vi "ISEG_HVChannel.ProcCases.vi"(0 "i ref in":refnum<vi>, 1 "selector":string, 2 "Data":T1, 3 "call cluster":T2={"Object"="", "Selector"="", "CallType"=enum."synchronous", "Async Object"="", "Async Selector"="", "Data Descriptor"="", "Data"=[], "Error #"=0, "Expire"=0}, 5 "error in (no error)":errorcluster) -> (14 "i ref out":refnum<vi>, 17 "answer cluster":T2={"Object"="", "Selector"="", "CallType"=enum."synchronous", "Async Object"="", "Async Selector"="", "Data Descriptor"="", "Data"=[], "Error #"=0, "Expire"=0}, 19 "error out":errorcluster)   [LabVIEW 2014, in "ISEG_HVChannel.lvlib"]
doc: "This method is called by a process from within the default case in the event loop. The methods of a class that are linked to events will be called from THIS method. Add your code here."
uses:
  ISEG_HVChannel.lvlib
  CS_Core/CSSystem/CoreDefs/CoreDefs.call_type.ctl
  CS_Core/BaseProcess/BaseProcess.descriptor string definition.ctl
  CS_Core/CSSystem/CoreDefs/CoreDefs.rawDataType.ctl
  CS_Core/CSApplicationBaseClasses/PSChannelBase/PSChannelBase.serviceType.ctl
  CS_Core/CSApplicationBaseClasses/PSChannelBase/PSChannelBase.directionType.ctl
  CSlibraries/UtilityLib/UtilityLib.valueStatus.ctl
  CS_Core/CSSystem/CoreDefs/CoreDefs.error_type.ctl
  CS_Core/CSSystem/CoreDefs/CoreDefs.error_severity.ctl
  CS_Core/CSSystem/CoreLib/CoreLib.string 2 byte array.vi
  CS_Core/CSSystem/CoreLib/CoreLib.byte array 2 int.vi
  CS_Core/CSSystem/CoreLib/CoreLib.byte array 2 double.vi
  CS_Core/CSSystem/CoreLib/CoreLib.double 2 byte array.vi
  CS_Core/CSSystem/CoreLib/CoreLib.short 2 byte array.vi
  CS_Core/CSSystem/CoreLib/CoreLib.byte array 2 short.vi
  CS_Core/CSSystem/CoreLib/CoreLib.lvlib
  CS_Core/BaseProcess/BaseProcess.lvlib
  CS_Core/CSApplicationBaseClasses/PSChannelBase/PSChannelBase.lvlib
  CSlibraries/UtilityLib/UtilityLib.lvlib
  CS_Core/CAEObj/CAEObj.lvlib
  CS_Core/CSApplicationBaseClasses/DeviceBase/DeviceBase.lvlib
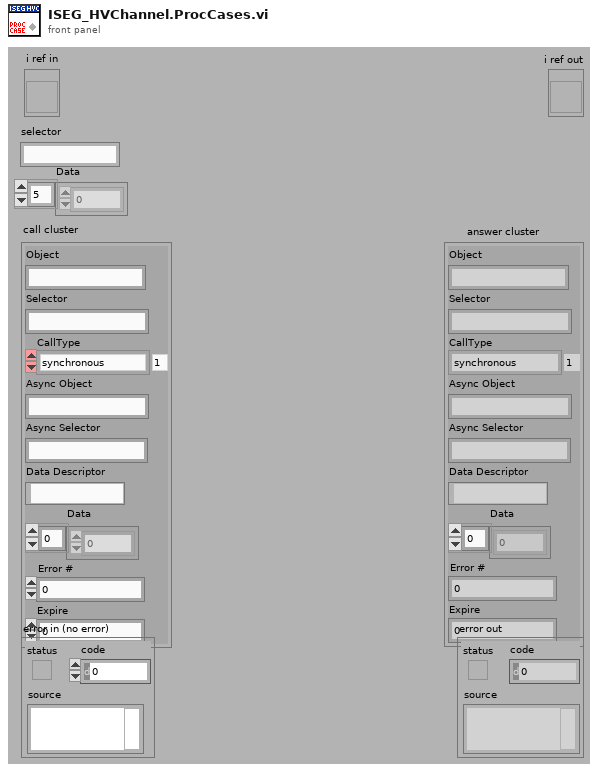
[diagram p1: front panel]
types:
  T1 = typedef "CoreDefs.rawDataType.ctl" = i8[]
  T2 = typedef "CoreDefs.call_type.ctl" = cluster{"Object":string, "Selector":string, "CallType":enum16{"simple", "synchronous", "asynchronous"}, "Async Object":string, "Async Selector":string, "Data Descriptor":T3, "Data":T1, "Error #":i32, "Expire":u32}
  T3 = typedef "BaseProcess.lvlib/BaseProcess.descriptor string definition.ctl" = string
  T4 = typedef "UtilityLib.lvlib/UtilityLib.valueStatus.ctl" = enum16{"no info available", "stand by/off", "on", "warning", "alarm/malfunction", "not implemented", "user action required", "important information", "system default", "control default", "indicator default", "button default"}
  T5 = typedef "PSChannelBase.lvlib/PSChannelBase.directionType.ctl" = enum16{"unknown", "update actual value", "update nominal value", "update both"}
  T6 = typedef "PSChannelBase.lvlib/PSChannelBase.serviceType.ctl" = enum16{"onOff", "voltage", "current", "tripCurrent", "rampUpSpeed", "rampDownSpeed", "status"}
  T7 = typedef "CoreDefs.error_severity.ctl" = enum16{"undefined", "information", "warning", "error", "fatal"}
  T8 = typedef "CoreDefs.error_type.ctl" = enum16{"no error", "can't load process", "can't unload process", "process does not exist", "can't install process", "can't remove process", "unknown function", "time out", "can't execute function", "duplicate queue name", "super not found", "caller queue invalid", "can't ping process", "unknown error", "VISA Error", "VISA timeout", "GPIB timeout", "GPIB error", "communication error", "data type mismatch", "can't read data from OPC server", "can't write data to OPC server", "OET error", "function not implemented", "process already exists", "invalid Shared Variable name", "error writing Shared Variable", "error reading Shared Variable", "invalid client name", "corrupt database", "unknown class", "call not authorized", "parameter out of range", "OET timeout: can't get data to modify", "invalid queue name", "requested operation incompatible with current state", "event undefined", "event disabled", "state undefined", "caller is not a friend", "EventBuilder: bad eventID", "EventBuilder: no DAQ devices", "a thread must not stop itself", "UNUSED ELEMENT4", "DiscArchiver: eventData incomplete", "DiscArchiver: eventData does not belong to run", "DiscArchiver: can't open file", "DiscArchiver: can't write to file", "DiscArchiver: available disc space low", "can't acquire semaphore", "error reading data from database", "notifier object is not existing", "can't register process", "can't unregister process", "illegal event type", "object disabled", "object already exists", "can't change state", "Instrument not found", "no connection to remote node", "invalid reference", "N/A", "UNUSED ELEMENT 1", "element not found", "illegal TCP/IP connection detected", "object does not exist", "invalid access ID", "unknown CS system", "invalid privilige", "unsupported data type", "unsupported server type", "IO server already exists", "Shared Variable already exists"}
  T9 = typedef "PSChannelBase.lvlib/PSChannelBase.i attribute.ctl" = cluster{"defaultChannelIndex":i32, "nofChannels":i32, "defaultChannelIndexID":i32, "nofChannelsID":i32, "actValues":T10, "nomValues":T10, "logicalName":string[], "physicalName":string[], "logicalNameID":i32, "physicalNameID":i32}
  T10 = typedef "PSChannelBase.lvlib/PSChannelBase.parameters.ctl" = cluster{"onOff":bool[], "voltage":dbl[], "current":dbl[], "tripCurrent":dbl[], "rampUpSpeed":dbl[], "rampDownSpeed":dbl[], "status":i32[], "serviceIDs":cluster{"onOfflID":i32, "voltageID":i32, "currentID":i32, "tripCurrentID":i32, "rampUpSpeedID":i32, "rampDownSpeedID":i32, "statusID":i32}}
  T11 = typedef "ISEG_HVChannel.lvlib/ISEG_HVChannel.i attribute.ctl" = cluster{"Channel Array":cluster{"Logical Name":string, "Address":string, "error in (no error)":errorcluster, "Status":cluster{"Status":i16, "DIM Status":T12}, "On":cluster{"On":bool, "DIM Status":T12}, "VMeas ":cluster{"VMeas":dbl, "DIM Status":T12}, "VSet ":cluster{"VSet":dbl, "DIM Status":T12}, "ITrip ":cluster{"ITrip":dbl, "DIM Status":T12}, "IMeas":cluster{"IMeas":dbl, "DIM Status":T12}, " RampSpeed":cluster{"RampSpeed":dbl, "DIM Status":T12}, "EventMask ":cluster{"EventMask":i16, "DIM Status":T12}}[], "VoltageInRangeBand":dbl, "NofCh":cluster{"NofCh":i32, "DIM Service":i32}, "BoardPrefix":string}
  T12 = typedef "ISEG_HVChannel.lvlib/ISEG_HVChannel.DIM Status.ctl" = cluster{"no link":bool, "quality":i32, "Time Stamp":timestamp}
  T13 = cluster{"Logical Name":string, "Address":string, "error in (no error)":errorcluster, "Status":cluster{"Status":i16, "DIM Status":T12}, "On":cluster{"On":bool, "DIM Status":T12}, "VMeas ":cluster{"VMeas":dbl, "DIM Status":T12}, "VSet ":cluster{"VSet":dbl, "DIM Status":T12}, "ITrip ":cluster{"ITrip":dbl, "DIM Status":T12}, "IMeas":cluster{"IMeas":dbl, "DIM Status":T12}, " RampSpeed":cluster{"RampSpeed":dbl, "DIM Status":T12}, "EventMask ":cluster{"EventMask":i16, "DIM Status":T12}}[]
  T14 = cluster{"Logical Name":string, "Address":string, "error in (no error)":errorcluster, "Status":cluster{"Status":i16, "DIM Status":T12}, "On":cluster{"On":bool, "DIM Status":T12}, "VMeas ":cluster{"VMeas":dbl, "DIM Status":T12}, "VSet ":cluster{"VSet":dbl, "DIM Status":T12}, "ITrip ":cluster{"ITrip":dbl, "DIM Status":T12}, "IMeas":cluster{"IMeas":dbl, "DIM Status":T12}, " RampSpeed":cluster{"RampSpeed":dbl, "DIM Status":T12}, "EventMask ":cluster{"EventMask":i16, "DIM Status":T12}}
  T15 = typedef "BaseProcess.lvlib/BaseProcess.i attribute.ctl" = cluster{"EventStatus":string, "EventError":i32, "PresetEvtWatchD":i32, "PresetPdcWatchD":i32, "EventTimeout":i32, "PeriodicInterval":i32, "Interface":string[], "Address":string[], "Special":string[], "PeriodicError":i32, "PeriodicStatus":string, "SuperProc":string, "Descriptors":T16[], "CaseRef":refnum<vi>, "PdcRef":refnum<vi>, "Thread Ref":refnum<vi>, "eventErrorID":i32, "eventStatusID":i32, "periodicErrorID":i32, "periodicStatusID":i32, "pdcCtrID":i32}
  T16 = typedef "BaseProcess.lvlib/BaseProcess.descriptor definition.ctl" = cluster{"selector":string, "descriptor":T3}
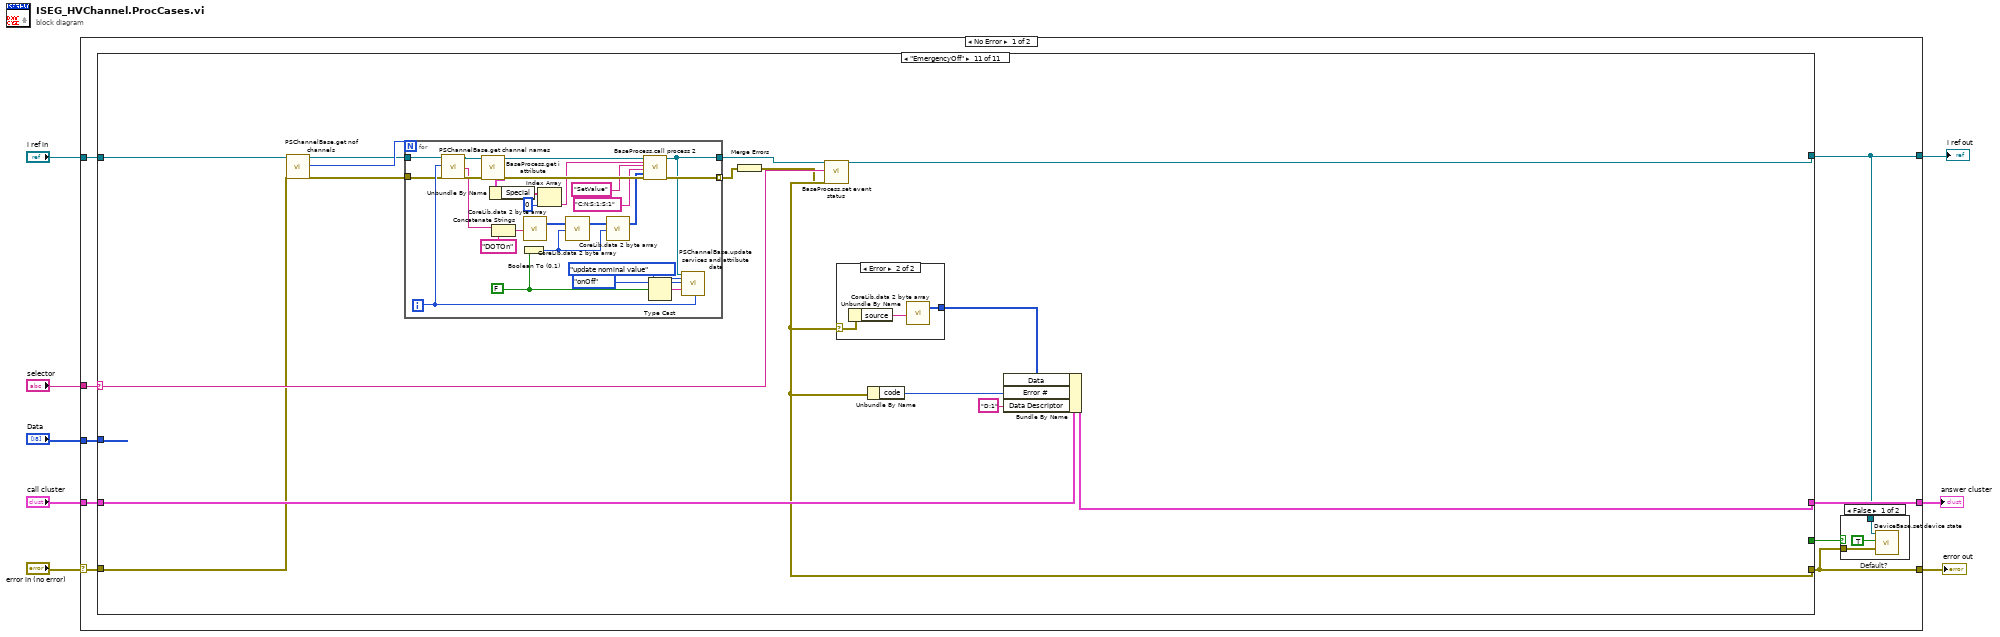
[diagram p0: block diagram]
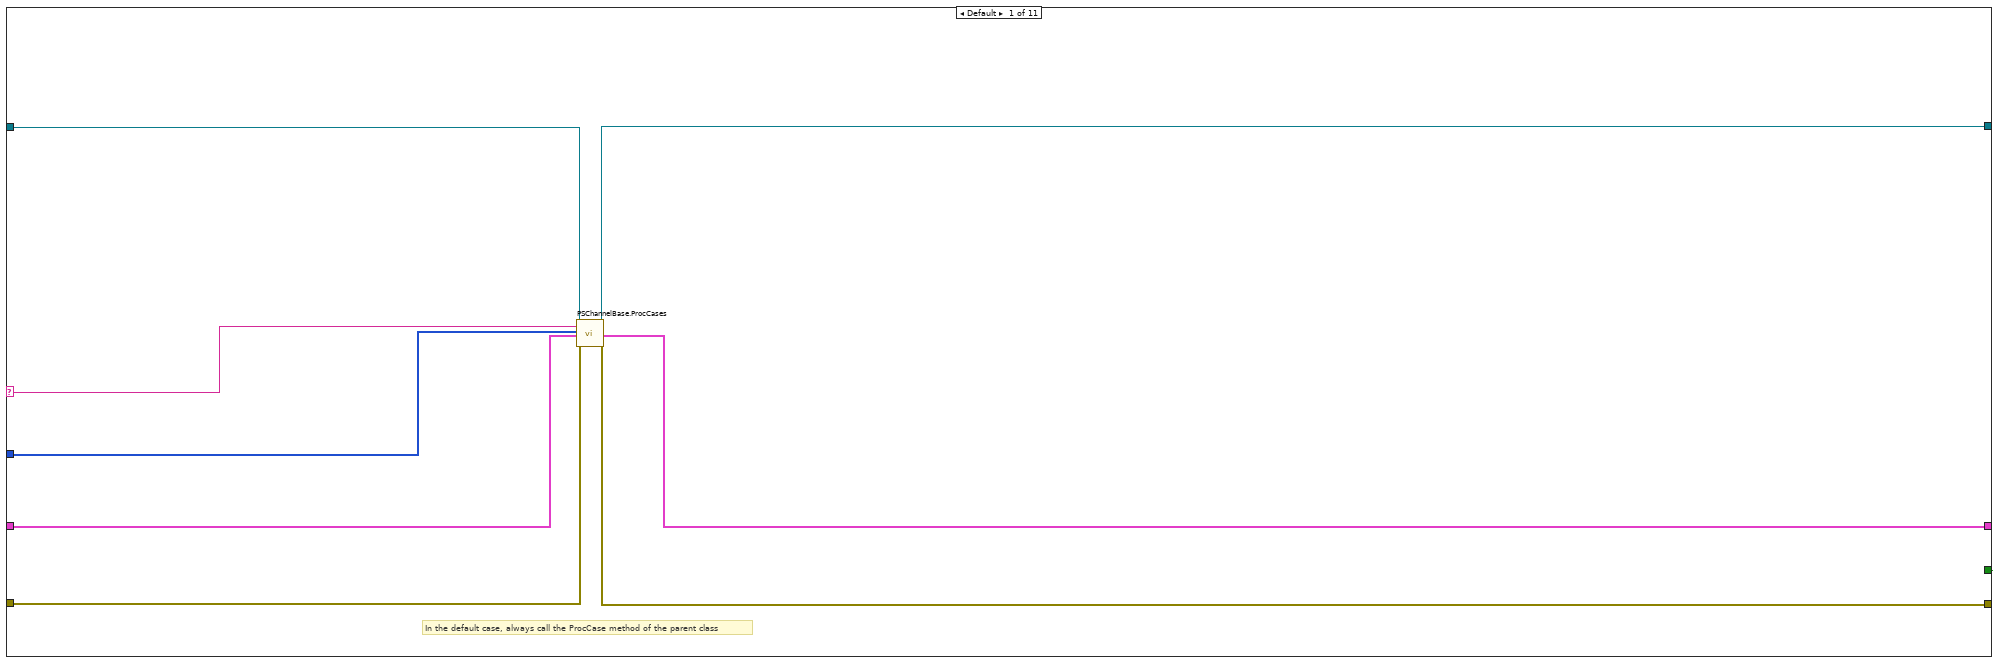
[diagram p3: hidden frame]
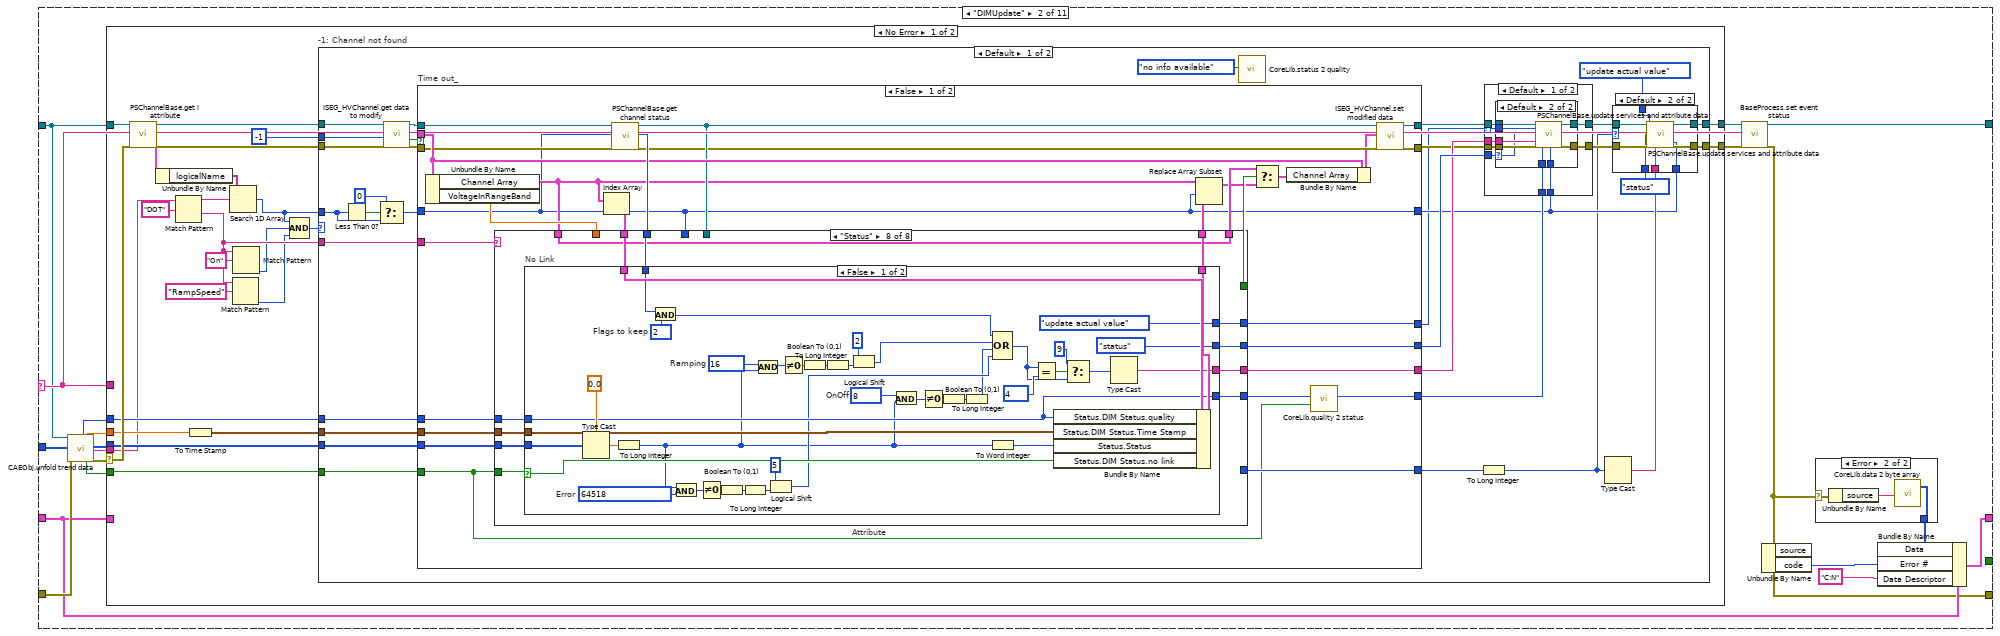
[diagram p4: hidden frame]
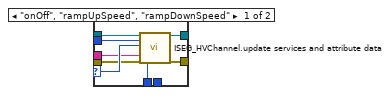
[diagram p6: hidden frame]
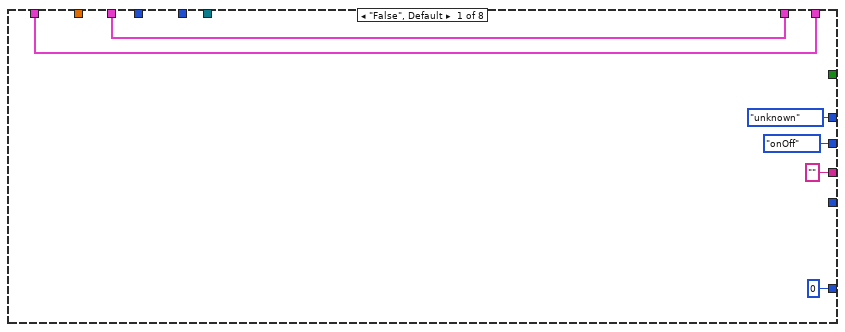
[diagram p9: hidden frame]
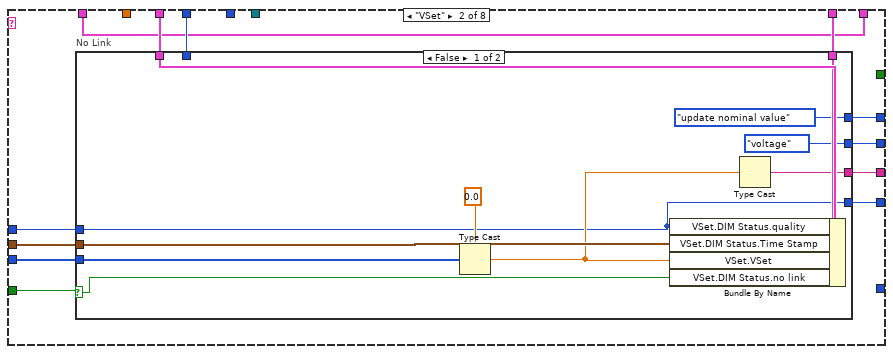
[diagram p10: hidden frame]
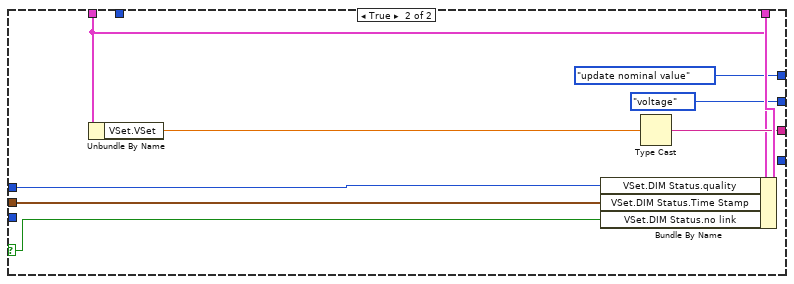
[diagram p11: hidden frame]
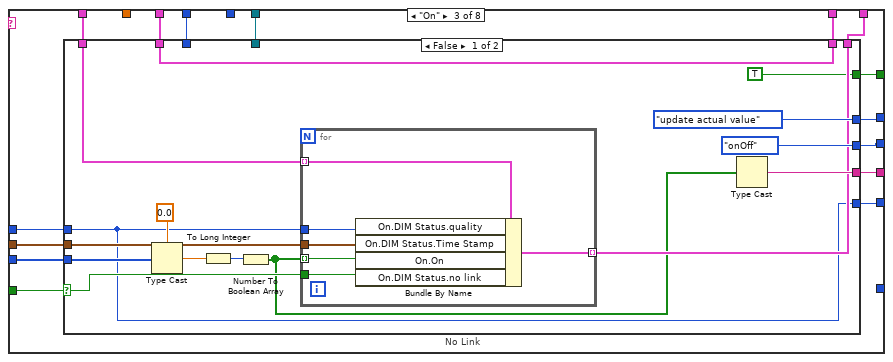
[diagram p12: hidden frame]
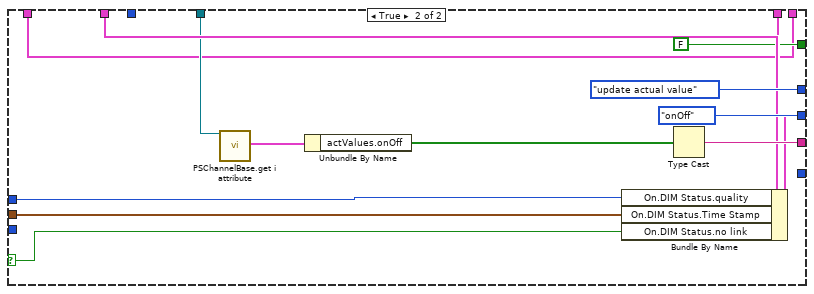
[diagram p13: hidden frame]
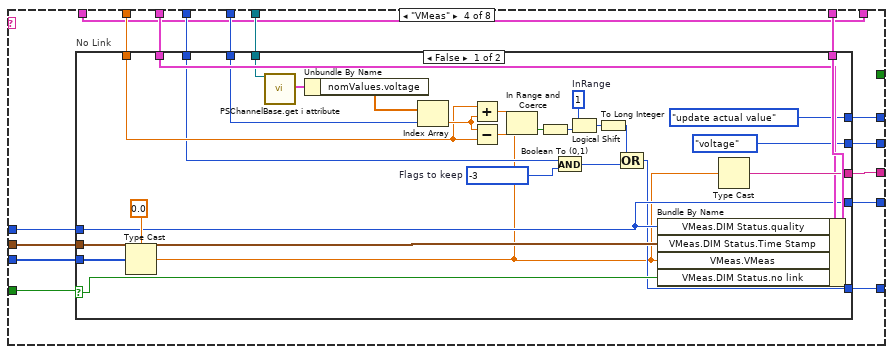
[diagram p14: hidden frame]
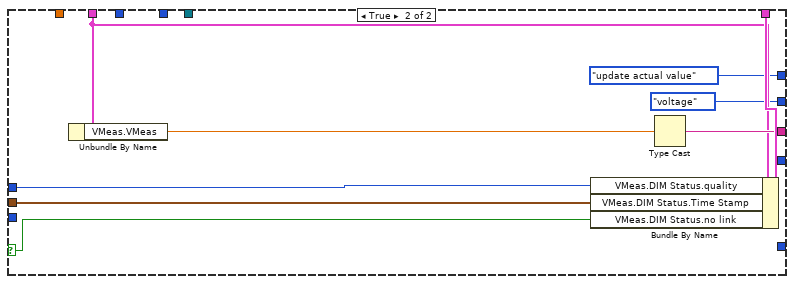
[diagram p15: hidden frame]
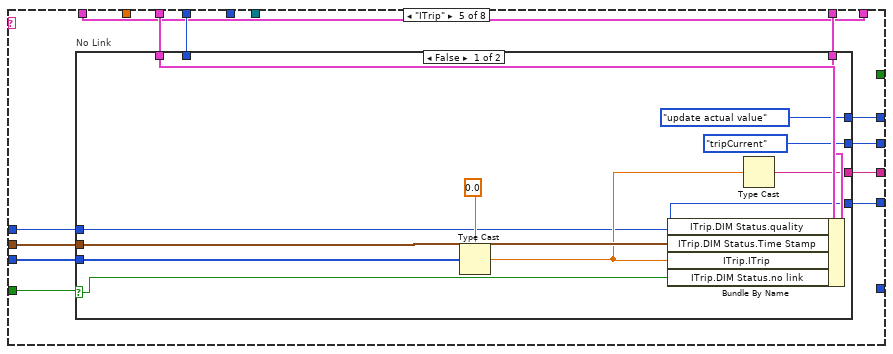
[diagram p16: hidden frame]
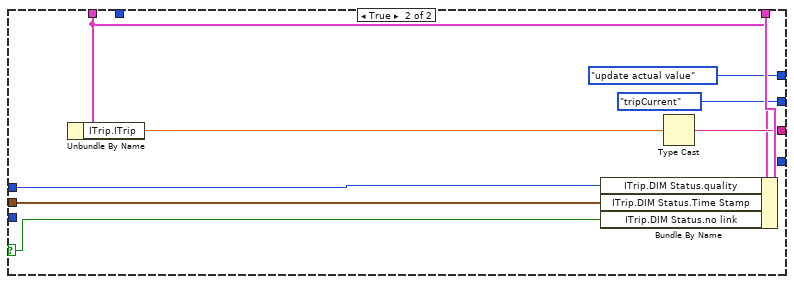
[diagram p17: hidden frame]
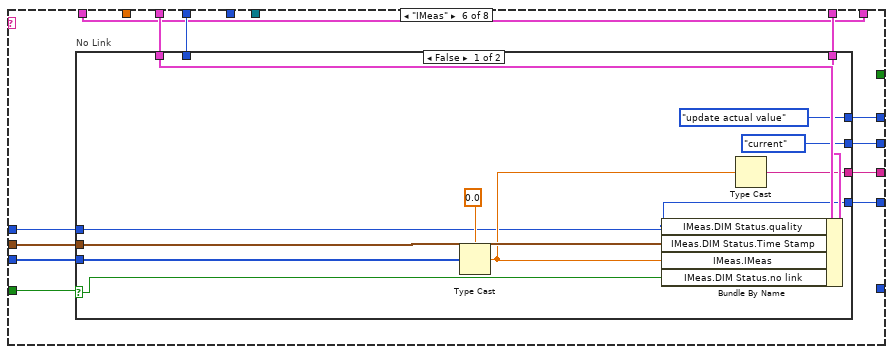
[diagram p18: hidden frame]
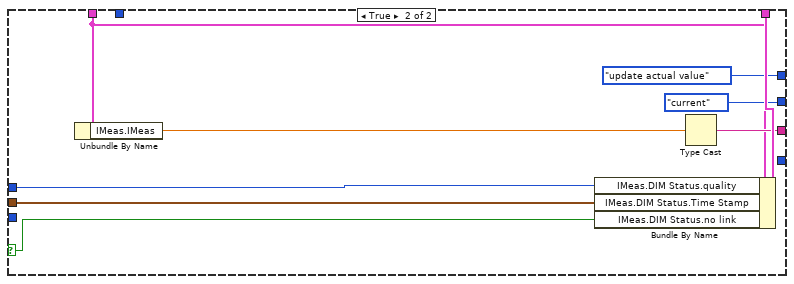
[diagram p19: hidden frame]
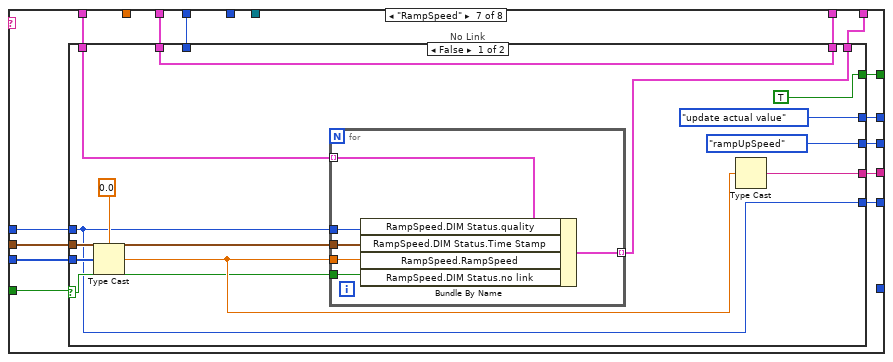
[diagram p20: hidden frame]
diagram:
  n1 = case shown="No Error" "error in (no error)" {
    selector: "error in (no error)" -> [w12 w963]
    tunnel: "selector" -> [w17 _]
    tunnel: [w16 w964] -> w7
    tunnel: "Data" -> [w15 _]
    tunnel: "call cluster" -> [w14 w964]
    tunnel: "i ref in" -> [w13 w965]
    tunnel: [w10 w965] -> w3
    tunnel: [w11 w963] -> w2
    frame No Error {
      n2 = case shown="\"EmergencyOff\"" w17 {
        selector: w17 -> [w24 w35 w511 w563 w610 w667 w721 w775 w829 w876 w927]
        tunnel: w15 -> [w22 w36 _ _ _ _ _ _ _ _ _]
        tunnel: w13 -> [w23 w30 w520 w556 w619 w658 w712 w766 w824 w885 w920]
        tunnel: [w29 w33 w510 w562 w609 w666 w720 w774 w828 w875 w926] -> w10
        tunnel: w14 -> [w25 w37 w517 w567 w616 w673 w727 w781 w835 w882 w931]
        tunnel: [w26 w34 w516 w566 w615 w672 w726 w780 w834 w881 w930] -> w16
        tunnel: w12 -> [w28 w38 w519 w557 w618 w675 w729 w783 w837 w884 w919]
        tunnel: [w27 w32 w512 w564 w611 w668 w722 w776 w830 w877 w928] -> w11
        tunnel: [TRUE _ _ _ _ _ _ _ _ _ _] -> w9
        frame Default {
          (unwired) TRUE
          # "In the default case, always call the ProcCase method of the parent class"
          n3 = call "PSChannelBase.ProcCases.vi"("i ref in"=w23, "selector"=w24, "Data"=w22, "call cluster"=w25, "error in (no error)"=w28) -> ("i ref out"=w29:refnum<vi>, "answer cluster"=w26:T2, "error out"=w27:errorcluster)  [unwired: 12 in]
        }
        frame "DIMUpdate" {
          n4 = call "CAEObj.unfold trend data.vi"("i ref in"=w30, "raw trend data"=w36, "error in (no error)"=w38) -> ("quality"=w48:i32, "timeStamp"=w47:dbl, "no link"=w43:bool, "data"=w46:i8[], "serviceName"=w45:string, "error out"=w44:errorcluster)  [unwired: 8 in, 3 out]
          n5 = case shown="No Error" w44 {
            selector: w44 -> [w74 w503]
            tunnel: w30 -> [w75 w501]
            tunnel: w48 -> [w67 _]
            tunnel: w47 -> [w66 _]
            tunnel: w46 -> [w64 _]
            tunnel: w45 -> [w60 _]
            tunnel: w43 -> [w63 _]
            tunnel: w37 -> [_ _]
            tunnel: w35 -> [_ _]
            tunnel: [w62 w502] -> w41
            tunnel: [w61 w501] -> w42
            frame No Error {
              n6 = call "PSChannelBase.get i attribute.vi"("i ref in"=w75, "error in (no error)"=w74) -> ("i ref out"=w70:refnum<vi>, "i attribute"=w71:T9, "error out"=w69:errorcluster)  [unwired: 15 in]
              n7 = Unbundle By Name(w71) -> ("logicalName"=w73:string[])
              n8 = Match Pattern(string=w60, regular expression="DOT") -> (before substring=w59:string, after substring=w58:string)  [unwired: 1 in, 2 out]
              n9 = To Time Stamp(1:w66) -> (0:w65:timestamp)
              n10 = Search 1D Array(1D array=w73, element=w59) -> (index of element=w55:i32)  [unwired: 1 in]
              n11 = Match Pattern(string=w58, regular expression="RampSpeed") -> (offset past match=w53:i32)  [unwired: 1 in, 3 out]
              n12 = Match Pattern(string=w58, regular expression="On") -> (offset past match=w54:i32)  [unwired: 1 in, 3 out]
              n13 = Compound Arithmetic op=AND(w55, w54, w53) -> (w52:i32)
              n14 = case "-1: Channel not found" shown="Default" w52 {
                tunnel: w70 -> [w108 w494]
                tunnel: w69 -> [w107 w495]
                tunnel: -1 -> [w106 _]
                tunnel: w58 -> [w101 _]
                tunnel: w67 -> [w100 _]
                tunnel: w65 -> [w99 _]
                tunnel: w64 -> [w98 _]
                tunnel: w63 -> [w97 _]
                tunnel: [w94 w494] -> w61
                tunnel: [w93 w493] -> w62
                tunnel: w55 -> [w80 _]
                frame Default {
                  n15 = Less Than 0?(x=w80) -> (x < 0?=w83:bool)
                  n16 = Select(t=0, s=w83, f=w80) -> (s? t:f=w82:i32)
                  n17 = call "ISEG_HVChannel.get data to modify.vi"("i ref in"=w108, "ms timeout (10000)"=w106, "error in (no error)"=w107) -> ("i ref out"=w105:refnum<vi>, "i attribute"=w104:T11, "timed out"=w102:bool, "error out"=w103:errorcluster)  [unwired: 13 in]
                  n18 = case "Time out_" shown="False" w102 {
                    tunnel: w105 -> [w174 w492]
                    tunnel: w104 -> [w168 _]
                    tunnel: w103 -> [w165 w491]
                    tunnel: w82 -> [w152 w490]
                    tunnel: w101 -> [w175 _]
                    tunnel: w100 -> [w169 _]
                    tunnel: w99 -> [w170 _]
                    tunnel: w98 -> [w171 _]
                    tunnel: w97 -> [w148 _]
                    tunnel: [w166 w492] -> w90
                    tunnel: [w163 w491] -> w79
                    tunnel: [w162 PSChannelBase.directionType."unknown" ("direction")] -> w78
                    tunnel: [w161 PSChannelBase.serviceType."onOff" ("service")] -> w89
                    tunnel: [w160 ""] -> w88
                    tunnel: [w152 w490] -> w86
                    tunnel: [w149 UtilityLib.valueStatus."no info available" ("valueStatus")] -> w87
                    tunnel: [w155 0] -> w96
                    frame False {
                      n19 = Unbundle By Name(w168) -> ("Channel Array"=w154:T13, "VoltageInRangeBand"=w156:dbl)
                      n20 = Index Array(array=w154, index=w152) -> (element=w172:T14)
                      n21 = call "PSChannelBase.get channel status.vi"("i ref in"=w174, "channelIndex"=w152, "error in (no error)"=w165) -> ("i ref out"=w167:refnum<vi>, "status"=w173:i32, "error out"=w164:errorcluster)  [unwired: 14 in]
                      n22 = case "Attribute" shown="\"Status\"" w175 {
                        tunnel: w173 -> [_ w188 w221 w272 w319 w352 w387 w427]
                        tunnel: w172 -> [w177 w193 w215 w278 w327 w359 w382 w435]
                        tunnel: w152 -> [_ _ _ w266 _ _ _ _]
                        tunnel: w167 -> [_ _ w217 w268 _ _ _ _]
                        tunnel: w148 -> [_ w192 w228 w277 w326 w358 w393 w434]
                        tunnel: w171 -> [_ w191 w227 w276 w325 w357 w392 w433]
                        tunnel: w170 -> [_ w190 w226 w275 w324 w356 w391 w432]
                        tunnel: w169 -> [_ w189 w225 w274 w323 w355 w390 w431]
                        tunnel: [PSChannelBase.directionType."unknown" ("direction") w187 w224 w270 w322 w354 w389 w430] -> w162
                        tunnel: [PSChannelBase.serviceType."onOff" ("service") w186 w223 w271 w321 w353 w388 w429] -> w161
                        tunnel: ["" w185 w222 w273 w320 w351 w386 w428] -> w160
                        tunnel: [_ w184 w218 w269 w318 w350 w385 w426] -> w147
                        tunnel: [w176 w182 w220 w263 w316 w348 w383 w424] -> w159
                        tunnel: [_ _ w219 _ _ _ w380 _] -> w158
                        tunnel: w156 -> [_ _ _ w267 _ _ _ _]
                        tunnel: [0 _ _ w265 _ _ _ _] -> w155
                        tunnel: w154 -> [w176 w182 w216 w263 w316 w348 w384 w424]
                        tunnel: [w177 w183 w214 w264 w317 w349 w381 w425] -> w153
                        frame "False", Default {
                        }
                        frame "VSet" {
                          n23 = case "No Link" shown="False" w192 {
                            selector: w192 -> [w201 w205]
                            tunnel: w193 -> [w204 w207]
                            tunnel: w191 -> [w200 _]
                            tunnel: w190 -> [w203 w212]
                            tunnel: w189 -> [w194 w213]
                            tunnel: [w202 w211] -> w183
                            tunnel: w188 -> [_ _]
                            tunnel: [PSChannelBase.directionType."update nominal value" ("direction") PSChannelBase.directionType."update nominal value" ("direction")] -> w187
                            tunnel: [PSChannelBase.serviceType."voltage" ("service") PSChannelBase.serviceType."voltage" ("service")] -> w186
                            tunnel: [w196 w208] -> w185
                            tunnel: [w194 _] -> w184
                            frame False {
                              n24 = Type Cast(type=0.0, x=w200) -> (*(type *) &x=w195:dbl)
                              n25 = Bundle By Name(cluster=w204, "VSet.DIM Status.quality"=w194, "VSet.DIM Status.Time Stamp"=w203, "VSet.VSet"=w195, "VSet.DIM Status.no link"=w201) -> (w202:T14)
                              n26 = Type Cast(x=w195) -> (*(type *) &x=w196:string)  [unwired: 1 in]
                            }
                            frame True {
                              n27 = Unbundle By Name(w207) -> ("VSet.VSet"=w206:dbl)
                              n28 = Bundle By Name(cluster=w207, "VSet.DIM Status.quality"=w213, "VSet.DIM Status.Time Stamp"=w212, "VSet.DIM Status.no link"=w205) -> (w211:T14)
                              n29 = Type Cast(x=w206) -> (*(type *) &x=w208:string)  [unwired: 1 in]
                            }
                          }
                        }
                        frame "On" {
                          n30 = case "No Link" shown="False" w228 {
                            selector: w228 -> [w242 w250]
                            tunnel: w215 -> [w229 w257]
                            tunnel: w227 -> [w241 _]
                            tunnel: w226 -> [w243 w261]
                            tunnel: w225 -> [w230 w262]
                            tunnel: [w234 w251] -> w220
                            tunnel: [PSChannelBase.directionType."update actual value" ("direction") PSChannelBase.directionType."update actual value" ("direction")] -> w224
                            tunnel: [PSChannelBase.serviceType."onOff" ("service") PSChannelBase.serviceType."onOff" ("service")] -> w223
                            tunnel: [w238 w258] -> w222
                            tunnel: w221 -> [_ _]
                            tunnel: [TRUE FALSE] -> w219
                            tunnel: w216 -> [w231 w251]
                            tunnel: [w230 _] -> w218
                            tunnel: w217 -> [_ w256]
                            tunnel: [w229 w253] -> w214
                            frame False {
                              n31 = Type Cast(type=0.0, x=w241) -> (*(type *) &x=w236:dbl)
                              n32 = To Long Integer(number=w236) -> (32bit integer=w235:i32)
                              n33 = Number To Boolean Array(number=w235) -> (Boolean array=w233:bool[])
                              n34 = for {
                                tunnel: w230 -> [w249]
                                tunnel: w243 -> [w248]
                                tunnel: w242 -> [w247]
                                tunnel: w233 -> [w246] mode=indexing
                                tunnel: [w245] -> w234 mode=indexing
                                tunnel: w231 -> [w244] mode=indexing
                                n35 = Bundle By Name(cluster=w244, "On.DIM Status.quality"=w249, "On.DIM Status.Time Stamp"=w248, "On.On"=w246, "On.DIM Status.no link"=w247) -> (w245:T14)
                              }
                              n36 = Type Cast(x=w233) -> (*(type *) &x=w238:string)  [unwired: 1 in]
                            }
                            frame True {
                              n37 = call "PSChannelBase.get i attribute.vi"("i ref in"=w256) -> ("i attribute"=w255:T9)  [unwired: 16 in, 2 out]
                              n38 = Unbundle By Name(w255) -> ("actValues.onOff"=w254:bool[])
                              n39 = Bundle By Name(cluster=w257, "On.DIM Status.quality"=w262, "On.DIM Status.Time Stamp"=w261, "On.DIM Status.no link"=w250) -> (w253:T14)
                              n40 = Type Cast(x=w254) -> (*(type *) &x=w258:string)  [unwired: 1 in]
                            }
                          }
                        }
                        frame "VMeas" {
                          n41 = case "No Link" shown="False" w277 {
                            selector: w277 -> [w304 w312]
                            tunnel: w278 -> [w300 w310]
                            tunnel: w276 -> [w303 _]
                            tunnel: w275 -> [w306 w314]
                            tunnel: w274 -> [w285 w315]
                            tunnel: [w305 w313] -> w264
                            tunnel: [w301 w311] -> w273
                            tunnel: w272 -> [w280 _]
                            tunnel: [PSChannelBase.serviceType."voltage" ("service") PSChannelBase.serviceType."voltage" ("service")] -> w271
                            tunnel: [PSChannelBase.directionType."update actual value" ("direction") PSChannelBase.directionType."update actual value" ("direction")] -> w270
                            tunnel: [w285 _] -> w269
                            tunnel: w268 -> [w299 _]
                            tunnel: w267 -> [w289 _]
                            tunnel: w266 -> [w288 _]
                            tunnel: [w282 _] -> w265
                            frame False {
                              w281 = -3  # Flags to keep
                              w293 = i16 1  # InRange
                              n42 = Type Cast(type=0.0, x=w303) -> (*(type *) &x=w279:dbl)
                              n43 = call "PSChannelBase.get i attribute.vi"("i ref in"=w299) -> ("i attribute"=w298:T9)  [unwired: 16 in, 2 out]
                              n44 = Unbundle By Name(w298) -> ("nomValues.voltage"=w297:dbl[])
                              n45 = Index Array(array=w297, index=w288) -> (element=w290:dbl)
                              n46 = Add(x=w289, y=w290) -> (x+y=w296:dbl)
                              n47 = Subtract(x=w290, y=w289) -> (x-y=w295:dbl)
                              n48 = In Range and Coerce(upper limit=w296, x=w279, lower limit=w295) -> (In Range?=w291:bool)  [unwired: 1 out]
                              n49 = Boolean To (0,1)(Boolean=w291) -> (0, 1=w294:i16)
                              n50 = And(x=w280, y=w281) -> (x .and. y?=w283:i32)
                              n51 = Logical Shift(y=w293, x=w294) -> (x << y=w292:i16)
                              n52 = To Long Integer(number=w292) -> (32bit integer=w284:i32)
                              n53 = Compound Arithmetic op=OR(w284, w283) -> (w282:i32)
                              n54 = Bundle By Name(cluster=w300, "VMeas.DIM Status.quality"=w285, "VMeas.DIM Status.Time Stamp"=w306, "VMeas.VMeas"=w279, "VMeas.DIM Status.no link"=w304) -> (w305:T14)
                              n55 = Type Cast(x=w279) -> (*(type *) &x=w301:string)  [unwired: 1 in]
                            }
                            frame True {
                              n56 = Unbundle By Name(w310) -> ("VMeas.VMeas"=w309:dbl)
                              n57 = Bundle By Name(cluster=w310, "VMeas.DIM Status.quality"=w315, "VMeas.DIM Status.Time Stamp"=w314, "VMeas.DIM Status.no link"=w312) -> (w313:T14)
                              n58 = Type Cast(x=w309) -> (*(type *) &x=w311:string)  [unwired: 1 in]
                            }
                          }
                        }
                        frame "ITrip" {
                          n59 = case "No Link" shown="False" w326 {
                            selector: w326 -> [w335 w344]
                            tunnel: w327 -> [w338 w340]
                            tunnel: w325 -> [w334 _]
                            tunnel: w324 -> [w337 w346]
                            tunnel: w323 -> [w328 w347]
                            tunnel: [w336 w345] -> w317
                            tunnel: [PSChannelBase.directionType."update actual value" ("direction") PSChannelBase.directionType."update actual value" ("direction")] -> w322
                            tunnel: [PSChannelBase.serviceType."tripCurrent" ("service") PSChannelBase.serviceType."tripCurrent" ("service")] -> w321
                            tunnel: [w330 w341] -> w320
                            tunnel: w319 -> [_ _]
                            tunnel: [w328 _] -> w318
                            frame False {
                              n60 = Type Cast(type=0.0, x=w334) -> (*(type *) &x=w329:dbl)
                              n61 = Bundle By Name(cluster=w338, "ITrip.DIM Status.quality"=w328, "ITrip.DIM Status.Time Stamp"=w337, "ITrip.ITrip"=w329, "ITrip.DIM Status.no link"=w335) -> (w336:T14)
                              n62 = Type Cast(x=w329) -> (*(type *) &x=w330:string)  [unwired: 1 in]
                            }
                            frame True {
                              n63 = Unbundle By Name(w340) -> ("ITrip.ITrip"=w339:dbl)
                              n64 = Bundle By Name(cluster=w340, "ITrip.DIM Status.quality"=w347, "ITrip.DIM Status.Time Stamp"=w346, "ITrip.DIM Status.no link"=w344) -> (w345:T14)
                              n65 = Type Cast(x=w339) -> (*(type *) &x=w341:string)  [unwired: 1 in]
                            }
                          }
                        }
                        frame "IMeas" {
                          n66 = case "No Link" shown="False" w358 {
                            selector: w358 -> [w367 w376]
                            tunnel: w359 -> [w370 w372]
                            tunnel: w357 -> [w366 _]
                            tunnel: w356 -> [w369 w378]
                            tunnel: w355 -> [w360 w379]
                            tunnel: [w368 w377] -> w349
                            tunnel: [PSChannelBase.directionType."update actual value" ("direction") PSChannelBase.directionType."update actual value" ("direction")] -> w354
                            tunnel: [PSChannelBase.serviceType."current" ("service") PSChannelBase.serviceType."current" ("service")] -> w353
                            tunnel: w352 -> [_ _]
                            tunnel: [w361 w373] -> w351
                            tunnel: [w360 _] -> w350
                            frame False {
                              n67 = Type Cast(type=0.0, x=w366) -> (*(type *) &x=w362:dbl)
                              n68 = Bundle By Name(cluster=w370, "IMeas.DIM Status.quality"=w360, "IMeas.DIM Status.Time Stamp"=w369, "IMeas.IMeas"=w362, "IMeas.DIM Status.no link"=w367) -> (w368:T14)
                              n69 = Type Cast(x=w362) -> (*(type *) &x=w361:string)  [unwired: 1 in]
                            }
                            frame True {
                              n70 = Unbundle By Name(w372) -> ("IMeas.IMeas"=w371:dbl)
                              n71 = Bundle By Name(cluster=w372, "IMeas.DIM Status.quality"=w379, "IMeas.DIM Status.Time Stamp"=w378, "IMeas.DIM Status.no link"=w376) -> (w377:T14)
                              n72 = Type Cast(x=w371) -> (*(type *) &x=w373:string)  [unwired: 1 in]
                            }
                          }
                        }
                        frame "RampSpeed" {
                          n73 = case "No Link" shown="False" w393 {
                            selector: w393 -> [w398 w421]
                            tunnel: w382 -> [w395 w414]
                            tunnel: w392 -> [w406 _]
                            tunnel: w391 -> [w400 w422]
                            tunnel: w390 -> [w396 w423]
                            tunnel: [PSChannelBase.directionType."update actual value" ("direction") PSChannelBase.directionType."update actual value" ("direction")] -> w389
                            tunnel: [PSChannelBase.serviceType."rampUpSpeed" ("service") PSChannelBase.serviceType."rampUpSpeed" ("service")] -> w388
                            tunnel: w387 -> [_ _]
                            tunnel: [w402 w418] -> w386
                            tunnel: [w396 _] -> w385
                            tunnel: w384 -> [w401 w416]
                            tunnel: [w397 w416] -> w383
                            tunnel: [w395 w417] -> w381
                            tunnel: [TRUE FALSE] -> w380
                            frame False {
                              n74 = Type Cast(type=0.0, x=w406) -> (*(type *) &x=w399:dbl)
                              n75 = for {
                                tunnel: [w412] -> w397 mode=indexing
                                tunnel: w401 -> [w411] mode=indexing
                                tunnel: w396 -> [w410]
                                tunnel: w400 -> [w409]
                                tunnel: w399 -> [w408]
                                tunnel: w398 -> [w407]
                                n76 = Bundle By Name(cluster=w411, "RampSpeed.DIM Status.quality"=w410, "RampSpeed.DIM Status.Time Stamp"=w409, "RampSpeed.RampSpeed"=w408, "RampSpeed.DIM Status.no link"=w407) -> (w412:T14)
                              }
                              n77 = Type Cast(x=w399) -> (*(type *) &x=w402:string)  [unwired: 1 in]
                            }
                            frame True {
                              n78 = Unbundle By Name(w414) -> ("RampSpeed.RampSpeed"=w413:dbl)
                              n79 = Bundle By Name(cluster=w414, "RampSpeed.DIM Status.quality"=w423, "RampSpeed.DIM Status.Time Stamp"=w422, "RampSpeed.DIM Status.no link"=w421) -> (w417:T14)
                              n80 = Type Cast(x=w413) -> (*(type *) &x=w418:string)  [unwired: 1 in]
                            }
                          }
                        }
                        frame "Status" {
                          n81 = case "No Link" shown="False" w434 {
                            selector: w434 -> [w472 w481]
                            tunnel: w435 -> [w475 w484]
                            tunnel: w433 -> [w471 _]
                            tunnel: w432 -> [w474 w483]
                            tunnel: w431 -> [w465 w476]
                            tunnel: [w473 w482] -> w425
                            tunnel: [PSChannelBase.directionType."update actual value" ("direction") PSChannelBase.directionType."update actual value" ("direction")] -> w430
                            tunnel: [PSChannelBase.serviceType."status" ("service") PSChannelBase.serviceType."status" ("service")] -> w429
                            tunnel: [w467 w480] -> w428
                            tunnel: w427 -> [w437 w477]
                            tunnel: [w465 _] -> w426
                            frame False {
                              w438 = 2  # Flags to keep
                              w450 = 16  # Ramping
                              w451 = 8  # OnOff
                              w459 = 64518  # Error
                              n82 = Type Cast(type=0.0, x=w471) -> (*(type *) &x=w464:dbl)
                              n83 = To Long Integer(number=w464) -> (32bit integer=w452:i32)
                              n84 = And(x=w437, y=w438) -> (x .and. y?=w436:i32)
                              n85 = And(x=w452, y=w459) -> (x .and. y?=w460:i32)
                              n86 = Not Equal To 0?(x=w460) -> (x != 0?=w462:bool)
                              n87 = Boolean To (0,1)(Boolean=w462) -> (0, 1=w463:i16)
                              n88 = To Long Integer(number=w463) -> (32bit integer=w458:i32)
                              n89 = And(x=w450, y=w452) -> (x .and. y?=w445:i32)
                              n90 = Logical Shift(y=5, x=w458) -> (x << y=w457:i32)
                              n91 = Not Equal To 0?(x=w445) -> (x != 0?=w448:bool)
                              n92 = Boolean To (0,1)(Boolean=w448) -> (0, 1=w449:i16)
                              n93 = To Long Integer(number=w449) -> (32bit integer=w446:i32)
                              n94 = Logical Shift(y=2, x=w446) -> (x << y=w444:i32)
                              n95 = And(x=w451, y=w452) -> (x .and. y?=w454:i32)
                              n96 = Not Equal To 0?(x=w454) -> (x != 0?=w455:bool)
                              n97 = Boolean To (0,1)(Boolean=w455) -> (0, 1=w456:i16)
                              n98 = To Long Integer(number=w456) -> (32bit integer=w453:i32)
                              n99 = To Word Integer(number=w452) -> (16bit integer=w466:i16)
                              n100 = Compound Arithmetic op=OR(w436, w444, w453, w457) -> (w441:i32)
                              n101 = Equal?(x=w441, y=4 ("OnOff")) -> (x = y?=w442:bool)
                              n102 = Bundle By Name(cluster=w475, "Status.DIM Status.quality"=w465, "Status.DIM Status.Time Stamp"=w474, "Status.Status"=w466, "Status.DIM Status.no link"=w472) -> (w473:T14)
                              n103 = Select(t=9, s=w442, f=w441) -> (s? t:f=w439:i32)
                              n104 = Type Cast(x=w439) -> (*(type *) &x=w467:string)  [unwired: 1 in]
                            }
                            frame True {
                              n105 = Bundle By Name(cluster=w484, "Status.DIM Status.quality"=w476, "Status.DIM Status.Time Stamp"=w483, "Status.DIM Status.no link"=w481) -> (w482:T14)
                              n106 = Type Cast(x=w477) -> (*(type *) &x=w480:string)  [unwired: 1 in]
                            }
                          }
                        }
                      }
                      n107 = Replace Array Subset(array=w154, new element=w153, index=w152) -> (w151:T13)
                      n108 = Select(t=w159, s=w158, f=w151) -> (s? t:f=w157:T13)
                      n109 = Bundle By Name(cluster=w168, "Channel Array"=w157) -> (w150:T11)
                      n110 = call "CoreLib.quality 2 status.vi"("quality"=w147, "NOLINK"=w148) -> ("valueStatus"=w149:T4)  [unwired: 17 in]
                      n111 = call "ISEG_HVChannel.set modified data.vi"("i ref in"=w167, "i attribute"=w150, "error in (no error)"=w164) -> ("i ref out"=w166:refnum<vi>, "error out"=w163:errorcluster)  [unwired: 15 in]
                    }
                    frame True {
                    }
                  }
                  n112 = call "CoreLib.status 2 quality.vi"("valueStatus"=UtilityLib.valueStatus."no info available") -> ()  [unwired: 18 in, 1 out]
                  n113 = To Long Integer(number=w96) -> (32bit integer=w76:i32)
                  n114 = case shown="Default" w78 {
                    selector: w78 -> [w109 _]
                    tunnel: w90 -> [w117 w136]
                    tunnel: w79 -> [w116 w135]
                    tunnel: w89 -> [w114 _]
                    tunnel: w88 -> [w115 _]
                    tunnel: w87 -> [w113 _]
                    tunnel: w86 -> [w112 _]
                    tunnel: [w111 w136] -> w85
                    tunnel: [w110 w135] -> w84
                    frame Default {
                      n115 = case shown="Default" w114 {
                        selector: w114 -> [w125 w128]
                        tunnel: w117 -> [w124 w134]
                        tunnel: w116 -> [w120 w131]
                        tunnel: w115 -> [w122 w130]
                        tunnel: w113 -> [w121 w126]
                        tunnel: w112 -> [_ w129]
                        tunnel: [w123 w133] -> w111
                        tunnel: [w119 w132] -> w110
                        tunnel: w109 -> [w118 w127]
                        frame "onOff", "rampUpSpeed", "rampDownSpeed" {
                          n116 = call "ISEG_HVChannel.update services and attribute data.vi"("i ref in"=w124, "direction"=w118, "service"=w125, "value"=w122, "error in (no error)"=w120, "quality"=w121) -> ("i ref out"=w123:refnum<vi>, "error out"=w119:errorcluster)  [unwired: 11 in, 1 out]
                        }
                        frame Default {
                          n117 = call "PSChannelBase.update services and attribute data.vi"("i ref in"=w134, "direction"=w127, "service"=w128, "value"=w130, "error in (no error)"=w131, "quality"=w126, "channelNumber"=w129) -> ("i ref out"=w133:refnum<vi>, "error out"=w132:errorcluster)  [unwired: 10 in, 1 out]
                        }
                      }
                    }
                    frame "unknown" {
                    }
                  }
                  n118 = Type Cast(x=w76) -> (*(type *) &x=w95:string)  [unwired: 1 in]
                  n119 = case shown="Default" w76 {
                    tunnel: [w138 w146] -> w94
                    tunnel: w85 -> [w138 w145]
                    tunnel: [w137 w143] -> w93
                    tunnel: w84 -> [w137 w144]
                    tunnel: w95 -> [_ w142]
                    tunnel: w86 -> [_ w139]
                    tunnel: PSChannelBase.directionType."update actual value" ("direction") -> [_ w141]
                    tunnel: PSChannelBase.serviceType."status" ("service") -> [_ w140]
                    frame 0 {
                    }
                    frame Default {
                      n120 = call "PSChannelBase.update services and attribute data.vi"("i ref in"=w145, "direction"=w141, "service"=w140, "value"=w142, "error in (no error)"=w144, "channelNumber"=w139) -> ("i ref out"=w146:refnum<vi>, "error out"=w143:errorcluster)  [unwired: 11 in, 1 out]
                    }
                  }
                }
                frame -1 {
                  n121 = call "CoreLib.my to LV error.vi"("ErrorTypes"=CoreDefs.error_type."element not found", "severityLevel"=CoreDefs.error_severity."warning") -> ("myErrorCluster"=w498:errorcluster)  [unwired: 16 in, 1 out]
                  n122 = Bundle By Name(cluster=w498, "source"="DIMUpdate") -> (w497:errorcluster)
                  n123 = Select(t=w495, s=w495, f=w497) -> (s? t:f=w493:errorcluster)
                }
              }
            }
            frame Error {
              n124 = call "CoreLib.set data type mismatch.vi"("error in (no error)"=w503) -> ("error out"=w502:errorcluster)  [unwired: 18 in]
            }
          }
          n125 = call "BaseProcess.set event status.vi"("i ref in"=w42, "EventStatus"=w35, "error in (no error)"=w41) -> ("i ref out"=w33:refnum<vi>, "error out"=w32:errorcluster)  [unwired: 14 in, 1 out]
          n126 = Unbundle By Name(w32) -> ("code"=w40:i32)  [unwired: 1 out]
          n127 = case shown="Error" w32 {
            selector: w32 -> [_ w51]
            tunnel: [_ w50] -> w31
            frame No Error {
            }
            frame Error {
              n128 = Unbundle By Name(w51) -> ("source"=w49:string)
              n129 = call-poly "CoreLib.data 2 byte array.vi"("string"=w49) -> ("byteArray out"=w50:T1)  [unwired: 18 in]
            }
          }
          n130 = Bundle By Name(cluster=w37, "Data"=w31, "Error #"=w40, "Data Descriptor"="C:N") -> (w34:T2)
        }
        frame "SetVoltage" {
          n131 = Unbundle By Name(w517) -> ("Data"=w506:T1)
          n132 = call-poly "CoreLib.byte array 2 data.vi"("byteArray"=w506) -> ("byteArray out"=w505:T1, "error out"=w504:errorcluster)  [unwired: 16 in, 1 out]
          n133 = call-poly "CoreLib.byte array 2 data.vi"("byteArray"=w505, "error in (no error)"=w504) -> ("d64"=w508:dbl, "error out"=w507:errorcluster)  [unwired: 15 in, 1 out]
          n134 = case shown="No Error" w507 {
            tunnel: [w527 w551] -> w514
            tunnel: w520 -> [w536 w551]
            tunnel: w519 -> [w535 w550]
            tunnel: [w528 w549] -> w513
            tunnel: w511 -> [_ w548]
            tunnel: w508 -> [w545 _]
            frame No Error {
              n135 = call "PSChannelBase.get default channel index.vi"("i ref in"=w536, "error in (no error)"=w535) -> ("i ref out"=w533:refnum<vi>, "defaultChannelIndex"=w526:i32, "error out"=w534:errorcluster)  [unwired: 15 in]
              n136 = call "PSChannelBase.get channel names.vi"("i ref in"=w533, "channelIndex"=w526, "error in (no error)"=w534) -> ("i ref out"=w532:refnum<vi>, "logicalName"=w525:string, "error out"=w531:errorcluster)  [unwired: 13 in, 1 out]
              n137 = Concatenate Strings(w525, "DOTVSet" ("string")) -> (w543:string)
              n138 = call "BaseProcess.get i attribute.vi"("i ref in"=w532, "error in (no error)"=w531) -> ("i ref out"=w530:refnum<vi>, "i attribute"=w540:T15, "error out"=w529:errorcluster)  [unwired: 15 in]
              n139 = Unbundle By Name(w540) -> ("Special"=w547:string[])
              n140 = call-poly "CoreLib.data 2 byte array.vi"("string"=w543) -> ("byteArray out"=w541:T1)  [unwired: 18 in]
              n141 = Index Array(array=w547, index=0) -> (element=w539:string)
              n142 = call-poly "CoreLib.data 2 byte array.vi"("byteArray"=w541, "f64"=w545) -> ("byteArray out"=w544:T1)  [unwired: 17 in]
              n143 = call "BaseProcess.call process 2.vi"("i ref in"=w530, "Object"=w539, "Selector"="SetValue", "Data Descriptor"="C:N;D:1;S:1", "Data"=w544, "error in (no error)"=w529) -> ("i ref out"=w527:refnum<vi>, "error out"=w528:errorcluster)  [unwired: 12 in]
            }
            frame Error {
              n144 = call "CoreLib.set data type mismatch.vi"("error in (no error)"=w550, "error source"=w548) -> ("error out"=w549:errorcluster)  [unwired: 17 in]
            }
          }
          n145 = call "BaseProcess.set event status.vi"("i ref in"=w514, "EventStatus"=w511, "error in (no error)"=w513) -> ("i ref out"=w510:refnum<vi>, "error out"=w512:errorcluster)  [unwired: 14 in, 1 out]
          n146 = case shown="Error" w512 {
            selector: w512 -> [_ w524]
            tunnel: [w521 w523] -> w515
            frame No Error {
              n147 = call-poly "CoreLib.data 2 byte array.vi"() -> ("byteArray out"=w521:T1)  [unwired: 19 in]
            }
            frame Error {
              n148 = Unbundle By Name(w524) -> ("source"=w522:string)
              n149 = call-poly "CoreLib.data 2 byte array.vi"("string"=w522) -> ("byteArray out"=w523:T1)  [unwired: 18 in]
            }
          }
          n150 = Unbundle By Name(w512) -> ("code"=w518:i32)
          n151 = Bundle By Name(cluster=w517, "Data"=w515, "Error #"=w518, "Data Descriptor"="D:1") -> (w516:T2)
        }
        frame "SetChannelRampUpSpeed" {
          n152 = Unbundle By Name(w567) -> ("Data"=w560:T1)
          n153 = call-poly "CoreLib.byte array 2 data.vi"("byteArray"=w560) -> ("byteArray out"=w559:T1, "error out"=w558:errorcluster)  [unwired: 16 in, 1 out]
          n154 = call-poly "CoreLib.byte array 2 data.vi"("byteArray"=w559, "error in (no error)"=w558) -> ("d64"=w555:dbl, "error out"=w554:errorcluster)  [unwired: 15 in, 1 out]
          n155 = case shown="No Error" w554 {
            tunnel: [w578 w598] -> w553
            tunnel: w556 -> [w576 w598]
            tunnel: w557 -> [w569 w597]
            tunnel: [w586 w596] -> w552
            tunnel: w555 -> [w577 _]
            frame No Error {
              n156 = call "ISEG_HVChannel.get i attribute.vi"("i ref in"=w576, "error in (no error)"=w569) -> ("i ref out"=w571:refnum<vi>, "i attribute"=w575:T11, "error out"=w570:errorcluster)  [unwired: 15 in]
              n157 = call "BaseProcess.get i attribute.vi"("i ref in"=w571, "error in (no error)"=w570) -> ("i ref out"=w588:refnum<vi>, "i attribute"=w592:T15, "error out"=w587:errorcluster)  [unwired: 15 in]
              n158 = Unbundle By Name(w575) -> ("BoardPrefix"=w574:string)
              n159 = Unbundle By Name(w592) -> ("Special"=w595:string[])
              n160 = Concatenate Strings(w574, "DOTRampSpeed" ("string")) -> (w572:string)
              n161 = call-poly "CoreLib.data 2 byte array.vi"("string"=w572) -> ("byteArray out"=w593:T1)  [unwired: 18 in]
              n162 = Index Array(array=w595, index=0) -> (element=w591:string)
              n163 = call-poly "CoreLib.data 2 byte array.vi"("byteArray"=w593, "f64"=w577) -> ("byteArray out"=w583:T1)  [unwired: 17 in]
              n164 = Boolean To (0,1)(Boolean=FALSE) -> (0, 1=w584:i16)
              n165 = call-poly "CoreLib.data 2 byte array.vi"("byteArray"=w583, "i16"=w584) -> ("byteArray out"=w582:T1)  [unwired: 17 in]
              n166 = call "BaseProcess.call process 2.vi"("i ref in"=w588, "Object"=w591, "Selector"="SetValue", "Data Descriptor"="C:N;D:1;S:1", "Data"=w582, "error in (no error)"=w587) -> ("i ref out"=w578:refnum<vi>, "error out"=w586:errorcluster)  [unwired: 12 in]
              n167 = Type Cast(x=w577) -> (*(type *) &x=w579:string)  [unwired: 1 in]
              n168 = call "PSChannelBase.update services and attribute data.vi"("i ref in"=w578, "direction"=PSChannelBase.directionType."update nominal value", "service"=PSChannelBase.serviceType."rampUpSpeed", "value"=w579) -> ()  [unwired: 13 in, 3 out]
            }
            frame Error {
              n169 = call "CoreLib.set data type mismatch.vi"("error in (no error)"=w597) -> ("error out"=w596:errorcluster)  [unwired: 18 in]
            }
          }
          n170 = call "BaseProcess.set event status.vi"("i ref in"=w553, "EventStatus"=w563, "error in (no error)"=w552) -> ("i ref out"=w562:refnum<vi>, "error out"=w564:errorcluster)  [unwired: 14 in, 1 out]
          n171 = case shown="Error" w564 {
            selector: w564 -> [_ w602]
            tunnel: [w599 w601] -> w565
            frame No Error {
              n172 = call-poly "CoreLib.data 2 byte array.vi"() -> ("byteArray out"=w599:T1)  [unwired: 19 in]
            }
            frame Error {
              n173 = Unbundle By Name(w602) -> ("source"=w600:string)
              n174 = call-poly "CoreLib.data 2 byte array.vi"("string"=w600) -> ("byteArray out"=w601:T1)  [unwired: 18 in]
            }
          }
          n175 = Unbundle By Name(w564) -> ("code"=w568:i32)
          n176 = Bundle By Name(cluster=w567, "Data"=w565, "Error #"=w568, "Data Descriptor"="D:1") -> (w566:T2)
        }
        frame "SetChannelRampDownSpeed" {
          n177 = Unbundle By Name(w616) -> ("Data"=w605:T1)
          n178 = call-poly "CoreLib.byte array 2 data.vi"("byteArray"=w605) -> ("byteArray out"=w607:T1, "error out"=w606:errorcluster)  [unwired: 16 in, 1 out]
          n179 = call-poly "CoreLib.byte array 2 data.vi"("byteArray"=w607, "error in (no error)"=w606) -> ("d64"=w603:dbl, "error out"=w604:errorcluster)  [unwired: 15 in, 1 out]
          n180 = case shown="No Error" w604 {
            tunnel: [w633 w654] -> w613
            tunnel: w619 -> [w631 w654]
            tunnel: w618 -> [w630 w653]
            tunnel: [w641 w652] -> w612
            tunnel: w610 -> [_ w651]
            tunnel: w603 -> [w632 _]
            frame No Error {
              n181 = call "ISEG_HVChannel.get i attribute.vi"("i ref in"=w631, "error in (no error)"=w630) -> ("i ref out"=w628:refnum<vi>, "i attribute"=w627:T11, "error out"=w629:errorcluster)  [unwired: 15 in]
              n182 = Unbundle By Name(w627) -> ("BoardPrefix"=w626:string)
              n183 = call "BaseProcess.get i attribute.vi"("i ref in"=w628, "error in (no error)"=w629) -> ("i ref out"=w643:refnum<vi>, "i attribute"=w647:T15, "error out"=w642:errorcluster)  [unwired: 15 in]
              n184 = Unbundle By Name(w647) -> ("Special"=w650:string[])
              n185 = Concatenate Strings(w626, "DOTRampSpeed" ("string")) -> (w624:string)
              n186 = Index Array(array=w650, index=0) -> (element=w646:string)
              n187 = call-poly "CoreLib.data 2 byte array.vi"("string"=w624) -> ("byteArray out"=w648:T1)  [unwired: 18 in]
              n188 = call-poly "CoreLib.data 2 byte array.vi"("byteArray"=w648, "f64"=w632) -> ("byteArray out"=w638:T1)  [unwired: 17 in]
              n189 = Boolean To (0,1)(Boolean=FALSE) -> (0, 1=w639:i16)
              n190 = call-poly "CoreLib.data 2 byte array.vi"("byteArray"=w638, "i16"=w639) -> ("byteArray out"=w637:T1)  [unwired: 17 in]
              n191 = call "BaseProcess.call process 2.vi"("i ref in"=w643, "Object"=w646, "Selector"="SetValue", "Data Descriptor"="C:N;D:1;S:1", "Data"=w637, "error in (no error)"=w642) -> ("i ref out"=w633:refnum<vi>, "error out"=w641:errorcluster)  [unwired: 12 in]
              n192 = Type Cast(x=w632) -> (*(type *) &x=w634:string)  [unwired: 1 in]
              n193 = call "PSChannelBase.update services and attribute data.vi"("i ref in"=w633, "direction"=PSChannelBase.directionType."update nominal value", "service"=PSChannelBase.serviceType."rampDownSpeed", "value"=w634) -> ()  [unwired: 13 in, 3 out]
            }
            frame Error {
              n194 = call "CoreLib.set data type mismatch.vi"("error in (no error)"=w653, "error source"=w651) -> ("error out"=w652:errorcluster)  [unwired: 17 in]
            }
          }
          n195 = call "BaseProcess.set event status.vi"("i ref in"=w613, "EventStatus"=w610, "error in (no error)"=w612) -> ("i ref out"=w609:refnum<vi>, "error out"=w611:errorcluster)  [unwired: 14 in, 1 out]
          n196 = case shown="Error" w611 {
            selector: w611 -> [_ w623]
            tunnel: [w620 w622] -> w614
            frame No Error {
              n197 = call-poly "CoreLib.data 2 byte array.vi"() -> ("byteArray out"=w620:T1)  [unwired: 19 in]
            }
            frame Error {
              n198 = Unbundle By Name(w623) -> ("source"=w621:string)
              n199 = call-poly "CoreLib.data 2 byte array.vi"("string"=w621) -> ("byteArray out"=w622:T1)  [unwired: 18 in]
            }
          }
          n200 = Unbundle By Name(w611) -> ("code"=w617:i32)
          n201 = Bundle By Name(cluster=w616, "Data"=w614, "Error #"=w617, "Data Descriptor"="D:1") -> (w615:T2)
        }
        frame "SetChannelVoltage" {
          n202 = Unbundle By Name(w673) -> ("Data"=w662:T1)
          n203 = call-poly "CoreLib.byte array 2 data.vi"("byteArray"=w662) -> ("byteArray out"=w661:T1, "i32"=w656:i32, "error out"=w660:errorcluster)  [unwired: 16 in]
          n204 = call "PSChannelBase.get channel names.vi"("i ref in"=w658, "channelIndex"=w656, "error in (no error)"=w660) -> ("i ref out"=w657:refnum<vi>, "logicalName"=w655:string, "error out"=w659:errorcluster)  [unwired: 13 in, 1 out]
          n205 = call-poly "CoreLib.byte array 2 data.vi"("byteArray"=w661, "error in (no error)"=w659) -> ("d64"=w664:dbl, "error out"=w663:errorcluster)  [unwired: 15 in, 1 out]
          n206 = case shown="No Error" w663 {
            tunnel: [w680 w708] -> w670
            tunnel: w657 -> [w690 w708]
            tunnel: w675 -> [w691 w707]
            tunnel: [w693 w706] -> w669
            tunnel: w667 -> [_ w705]
            tunnel: w664 -> [w686 _]
            tunnel: w655 -> [w692 _]
            tunnel: w656 -> [w685 _]
            frame No Error {
              n207 = Concatenate Strings(w692, "DOTVSet" ("string")) -> (w702:string)
              n208 = call "BaseProcess.get i attribute.vi"("i ref in"=w690, "error in (no error)"=w691) -> ("i ref out"=w695:refnum<vi>, "i attribute"=w699:T15, "error out"=w694:errorcluster)  [unwired: 15 in]
              n209 = Unbundle By Name(w699) -> ("Special"=w704:string[])
              n210 = call-poly "CoreLib.data 2 byte array.vi"("string"=w702) -> ("byteArray out"=w700:T1)  [unwired: 18 in]
              n211 = Index Array(array=w704, index=0) -> (element=w698:string)
              n212 = call-poly "CoreLib.data 2 byte array.vi"("byteArray"=w700, "f64"=w686) -> ("byteArray out"=w684:T1)  [unwired: 17 in]
              n213 = Boolean To (0,1)(Boolean=FALSE) -> (0, 1=w681:i16)
              n214 = call-poly "CoreLib.data 2 byte array.vi"("byteArray"=w684, "i16"=w681) -> ("byteArray out"=w683:T1)  [unwired: 17 in]
              n215 = call "BaseProcess.call process 2.vi"("i ref in"=w695, "Object"=w698, "Selector"="SetValue", "Data Descriptor"="C:N;D:1;S:1", "Data"=w683, "error in (no error)"=w694) -> ("i ref out"=w680:refnum<vi>, "error out"=w693:errorcluster)  [unwired: 12 in]
              n216 = Type Cast(x=w686) -> (*(type *) &x=w687:string)  [unwired: 1 in]
              n217 = call "PSChannelBase.update services and attribute data.vi"("i ref in"=w680, "direction"=PSChannelBase.directionType."update nominal value", "service"=PSChannelBase.serviceType."voltage", "value"=w687, "channelNumber"=w685) -> ()  [unwired: 12 in, 3 out]
            }
            frame Error {
              n218 = call "CoreLib.set data type mismatch.vi"("error in (no error)"=w707, "error source"=w705) -> ("error out"=w706:errorcluster)  [unwired: 17 in]
            }
          }
          n219 = call "BaseProcess.set event status.vi"("i ref in"=w670, "EventStatus"=w667, "error in (no error)"=w669) -> ("i ref out"=w666:refnum<vi>, "error out"=w668:errorcluster)  [unwired: 14 in, 1 out]
          n220 = case shown="No Error" w668 {
            selector: w668 -> [_ w679]
            tunnel: [w676 w678] -> w671
            frame No Error {
              n221 = call-poly "CoreLib.data 2 byte array.vi"() -> ("byteArray out"=w676:T1)  [unwired: 19 in]
            }
            frame Error {
              n222 = Unbundle By Name(w679) -> ("source"=w677:string)
              n223 = call-poly "CoreLib.data 2 byte array.vi"("string"=w677) -> ("byteArray out"=w678:T1)  [unwired: 18 in]
            }
          }
          n224 = Unbundle By Name(w668) -> ("code"=w674:i32)
          n225 = Bundle By Name(cluster=w673, "Data"=w671, "Error #"=w674, "Data Descriptor"="D:1") -> (w672:T2)
        }
        frame "SetChannelCurrent" {
          n226 = Unbundle By Name(w727) -> ("Data"=w716:T1)
          n227 = call-poly "CoreLib.byte array 2 data.vi"("byteArray"=w716) -> ("byteArray out"=w715:T1, "i32"=w710:i32, "error out"=w714:errorcluster)  [unwired: 16 in]
          n228 = call "PSChannelBase.get channel names.vi"("i ref in"=w712, "channelIndex"=w710, "error in (no error)"=w714) -> ("i ref out"=w711:refnum<vi>, "logicalName"=w709:string, "error out"=w713:errorcluster)  [unwired: 13 in, 1 out]
          n229 = call-poly "CoreLib.byte array 2 data.vi"("byteArray"=w715, "error in (no error)"=w713) -> ("d64"=w718:dbl, "error out"=w717:errorcluster)  [unwired: 15 in, 1 out]
          n230 = case shown="No Error" w717 {
            tunnel: [w734 w762] -> w724
            tunnel: w711 -> [w744 w762]
            tunnel: w729 -> [w745 w761]
            tunnel: [w747 w760] -> w723
            tunnel: w721 -> [_ w759]
            tunnel: w718 -> [w740 _]
            tunnel: w709 -> [w746 _]
            tunnel: w710 -> [w739 _]
            frame No Error {
              n231 = Concatenate Strings(w746, "DOTISet" ("string")) -> (w756:string)
              n232 = call "BaseProcess.get i attribute.vi"("i ref in"=w744, "error in (no error)"=w745) -> ("i ref out"=w749:refnum<vi>, "i attribute"=w753:T15, "error out"=w748:errorcluster)  [unwired: 15 in]
              n233 = Unbundle By Name(w753) -> ("Special"=w758:string[])
              n234 = call-poly "CoreLib.data 2 byte array.vi"("string"=w756) -> ("byteArray out"=w754:T1)  [unwired: 18 in]
              n235 = Index Array(array=w758, index=0) -> (element=w752:string)
              n236 = call-poly "CoreLib.data 2 byte array.vi"("byteArray"=w754, "f64"=w740) -> ("byteArray out"=w738:T1)  [unwired: 17 in]
              n237 = Boolean To (0,1)(Boolean=FALSE) -> (0, 1=w735:i16)
              n238 = call-poly "CoreLib.data 2 byte array.vi"("byteArray"=w738, "i16"=w735) -> ("byteArray out"=w737:T1)  [unwired: 17 in]
              n239 = call "BaseProcess.call process 2.vi"("i ref in"=w749, "Object"=w752, "Selector"="SetValue", "Data Descriptor"="C:N;D:1;S:1", "Data"=w737, "error in (no error)"=w748) -> ("i ref out"=w734:refnum<vi>, "error out"=w747:errorcluster)  [unwired: 12 in]
              n240 = Type Cast(x=w740) -> (*(type *) &x=w741:string)  [unwired: 1 in]
              n241 = call "PSChannelBase.update services and attribute data.vi"("i ref in"=w734, "direction"=PSChannelBase.directionType."update nominal value", "service"=PSChannelBase.serviceType."current", "value"=w741, "channelNumber"=w739) -> ()  [unwired: 12 in, 3 out]
            }
            frame Error {
              n242 = call "CoreLib.set data type mismatch.vi"("error in (no error)"=w761, "error source"=w759) -> ("error out"=w760:errorcluster)  [unwired: 17 in]
            }
          }
          n243 = call "BaseProcess.set event status.vi"("i ref in"=w724, "EventStatus"=w721, "error in (no error)"=w723) -> ("i ref out"=w720:refnum<vi>, "error out"=w722:errorcluster)  [unwired: 14 in, 1 out]
          n244 = case shown="No Error" w722 {
            selector: w722 -> [_ w733]
            tunnel: [w730 w732] -> w725
            frame No Error {
              n245 = call-poly "CoreLib.data 2 byte array.vi"() -> ("byteArray out"=w730:T1)  [unwired: 19 in]
            }
            frame Error {
              n246 = Unbundle By Name(w733) -> ("source"=w731:string)
              n247 = call-poly "CoreLib.data 2 byte array.vi"("string"=w731) -> ("byteArray out"=w732:T1)  [unwired: 18 in]
            }
          }
          n248 = Unbundle By Name(w722) -> ("code"=w728:i32)
          n249 = Bundle By Name(cluster=w727, "Data"=w725, "Error #"=w728, "Data Descriptor"="D:1") -> (w726:T2)
        }
        frame "SetChannelTripCurrent" {
          n250 = Unbundle By Name(w781) -> ("Data"=w770:T1)
          n251 = call-poly "CoreLib.byte array 2 data.vi"("byteArray"=w770) -> ("byteArray out"=w769:T1, "i32"=w764:i32, "error out"=w768:errorcluster)  [unwired: 16 in]
          n252 = call "PSChannelBase.get channel names.vi"("i ref in"=w766, "channelIndex"=w764, "error in (no error)"=w768) -> ("i ref out"=w765:refnum<vi>, "logicalName"=w763:string, "error out"=w767:errorcluster)  [unwired: 13 in, 1 out]
          n253 = call-poly "CoreLib.byte array 2 data.vi"("byteArray"=w769, "error in (no error)"=w767) -> ("d64"=w772:dbl, "error out"=w771:errorcluster)  [unwired: 15 in, 1 out]
          n254 = case shown="No Error" w771 {
            tunnel: [w788 w816] -> w778
            tunnel: w765 -> [w798 w816]
            tunnel: w783 -> [w799 w815]
            tunnel: [w801 w814] -> w777
            tunnel: w775 -> [_ w813]
            tunnel: w772 -> [w794 _]
            tunnel: w763 -> [w800 _]
            tunnel: w764 -> [w793 _]
            frame No Error {
              n255 = Concatenate Strings(w800, "DOTITrip" ("string")) -> (w810:string)
              n256 = call "BaseProcess.get i attribute.vi"("i ref in"=w798, "error in (no error)"=w799) -> ("i ref out"=w803:refnum<vi>, "i attribute"=w807:T15, "error out"=w802:errorcluster)  [unwired: 15 in]
              n257 = Unbundle By Name(w807) -> ("Special"=w812:string[])
              n258 = call-poly "CoreLib.data 2 byte array.vi"("string"=w810) -> ("byteArray out"=w808:T1)  [unwired: 18 in]
              n259 = Index Array(array=w812, index=0) -> (element=w806:string)
              n260 = call-poly "CoreLib.data 2 byte array.vi"("byteArray"=w808, "f64"=w794) -> ("byteArray out"=w792:T1)  [unwired: 17 in]
              n261 = Boolean To (0,1)(Boolean=FALSE) -> (0, 1=w789:i16)
              n262 = call-poly "CoreLib.data 2 byte array.vi"("byteArray"=w792, "i16"=w789) -> ("byteArray out"=w791:T1)  [unwired: 17 in]
              n263 = call "BaseProcess.call process 2.vi"("i ref in"=w803, "Object"=w806, "Selector"="SetValue", "Data Descriptor"="C:N;D:1;S:1", "Data"=w791, "error in (no error)"=w802) -> ("i ref out"=w788:refnum<vi>, "error out"=w801:errorcluster)  [unwired: 12 in]
              n264 = Type Cast(x=w794) -> (*(type *) &x=w795:string)  [unwired: 1 in]
              n265 = call "PSChannelBase.update services and attribute data.vi"("i ref in"=w788, "direction"=PSChannelBase.directionType."update nominal value", "service"=PSChannelBase.serviceType."tripCurrent", "value"=w795, "channelNumber"=w793) -> ()  [unwired: 12 in, 3 out]
            }
            frame Error {
              n266 = call "CoreLib.set data type mismatch.vi"("error in (no error)"=w815, "error source"=w813) -> ("error out"=w814:errorcluster)  [unwired: 17 in]
            }
          }
          n267 = call "BaseProcess.set event status.vi"("i ref in"=w778, "EventStatus"=w775, "error in (no error)"=w777) -> ("i ref out"=w774:refnum<vi>, "error out"=w776:errorcluster)  [unwired: 14 in, 1 out]
          n268 = case shown="No Error" w776 {
            selector: w776 -> [_ w787]
            tunnel: [w784 w786] -> w779
            frame No Error {
              n269 = call-poly "CoreLib.data 2 byte array.vi"() -> ("byteArray out"=w784:T1)  [unwired: 19 in]
            }
            frame Error {
              n270 = Unbundle By Name(w787) -> ("source"=w785:string)
              n271 = call-poly "CoreLib.data 2 byte array.vi"("string"=w785) -> ("byteArray out"=w786:T1)  [unwired: 18 in]
            }
          }
          n272 = Unbundle By Name(w776) -> ("code"=w782:i32)
          n273 = Bundle By Name(cluster=w781, "Data"=w779, "Error #"=w782, "Data Descriptor"="D:1") -> (w780:T2)
        }
        frame "SetChannelOnOff" {
          n274 = Unbundle By Name(w835) -> ("Data"=w826:T1)
          n275 = call-poly "CoreLib.byte array 2 data.vi"("byteArray"=w826) -> ("byteArray out"=w820:T1, "i32"=w822:i32, "error out"=w825:errorcluster)  [unwired: 16 in]
          n276 = call "PSChannelBase.get channel names.vi"("i ref in"=w824, "channelIndex"=w822, "error in (no error)"=w825) -> ("i ref out"=w823:refnum<vi>, "logicalName"=w821:string, "error out"=w819:errorcluster)  [unwired: 13 in, 1 out]
          n277 = call-poly "CoreLib.byte array 2 data.vi"("byteArray"=w820, "error in (no error)"=w819) -> ("i16"=w818:i16, "error out"=w817:errorcluster)  [unwired: 15 in, 1 out]
          n278 = case shown="No Error" w817 {
            tunnel: [w845 w870] -> w832
            tunnel: w823 -> [w853 w870]
            tunnel: w837 -> [w854 w869]
            tunnel: [w856 w868] -> w831
            tunnel: w829 -> [_ w867]
            tunnel: w818 -> [w844 _]
            tunnel: w821 -> [w855 _]
            tunnel: w822 -> [w849 _]
            frame No Error {
              n279 = Concatenate Strings(w855, "DOTOn" ("string")) -> (w864:string)
              n280 = call "BaseProcess.get i attribute.vi"("i ref in"=w853, "error in (no error)"=w854) -> ("i ref out"=w858:refnum<vi>, "i attribute"=w862:T15, "error out"=w857:errorcluster)  [unwired: 15 in]
              n281 = Unbundle By Name(w862) -> ("Special"=w866:string[])
              n282 = call-poly "CoreLib.data 2 byte array.vi"("string"=w864) -> ("byteArray out"=w843:T1)  [unwired: 18 in]
              n283 = Index Array(array=w866, index=0) -> (element=w861:string)
              n284 = Boolean To (0,1)(Boolean=FALSE) -> (0, 1=w846:i16)
              n285 = call-poly "CoreLib.data 2 byte array.vi"("byteArray"=w843, "i16"=w844) -> ("byteArray out"=w842:T1)  [unwired: 17 in]
              n286 = call-poly "CoreLib.data 2 byte array.vi"("byteArray"=w842, "i16"=w846) -> ("byteArray out"=w848:T1)  [unwired: 17 in]
              n287 = call "BaseProcess.call process 2.vi"("i ref in"=w858, "Object"=w861, "Selector"="SetValue", "Data Descriptor"="C:N;S:1;S:1", "Data"=w848, "error in (no error)"=w857) -> ("i ref out"=w845:refnum<vi>, "error out"=w856:errorcluster)  [unwired: 12 in]
              n288 = Type Cast(x=w844) -> (*(type *) &x=w850:string)  [unwired: 1 in]
              n289 = call "PSChannelBase.update services and attribute data.vi"("i ref in"=w845, "direction"=PSChannelBase.directionType."update nominal value", "service"=PSChannelBase.serviceType."onOff", "value"=w850, "channelNumber"=w849) -> ()  [unwired: 12 in, 3 out]
            }
            frame Error {
              n290 = call "CoreLib.set data type mismatch.vi"("error in (no error)"=w869, "error source"=w867) -> ("error out"=w868:errorcluster)  [unwired: 17 in]
            }
          }
          n291 = call "BaseProcess.set event status.vi"("i ref in"=w832, "EventStatus"=w829, "error in (no error)"=w831) -> ("i ref out"=w828:refnum<vi>, "error out"=w830:errorcluster)  [unwired: 14 in, 1 out]
          n292 = case shown="No Error" w830 {
            selector: w830 -> [_ w841]
            tunnel: [w838 w840] -> w833
            frame No Error {
              n293 = call-poly "CoreLib.data 2 byte array.vi"() -> ("byteArray out"=w838:T1)  [unwired: 19 in]
            }
            frame Error {
              n294 = Unbundle By Name(w841) -> ("source"=w839:string)
              n295 = call-poly "CoreLib.data 2 byte array.vi"("string"=w839) -> ("byteArray out"=w840:T1)  [unwired: 18 in]
            }
          }
          n296 = Unbundle By Name(w830) -> ("code"=w836:i32)
          n297 = Bundle By Name(cluster=w835, "Data"=w833, "Error #"=w836, "Data Descriptor"="D:1") -> (w834:T2)
        }
        frame "SetOnOff" {
          n298 = Unbundle By Name(w882) -> ("Data"=w873:T1)
          n299 = call-poly "CoreLib.byte array 2 data.vi"("byteArray"=w873) -> ("i16"=w872:i16, "error out"=w871:errorcluster)  [unwired: 16 in, 1 out]
          n300 = case shown="No Error" w871 {
            tunnel: [w892 w916] -> w879
            tunnel: w885 -> [w901 w916]
            tunnel: w884 -> [w900 w915]
            tunnel: [w893 w914] -> w878
            tunnel: w876 -> [_ w913]
            tunnel: w872 -> [w910 _]
            frame No Error {
              n301 = call "PSChannelBase.get default channel index.vi"("i ref in"=w901, "error in (no error)"=w900) -> ("i ref out"=w898:refnum<vi>, "defaultChannelIndex"=w891:i32, "error out"=w899:errorcluster)  [unwired: 15 in]
              n302 = call "PSChannelBase.get channel names.vi"("i ref in"=w898, "channelIndex"=w891, "error in (no error)"=w899) -> ("i ref out"=w897:refnum<vi>, "logicalName"=w890:string, "error out"=w896:errorcluster)  [unwired: 13 in, 1 out]
              n303 = Concatenate Strings(w890, "DOTOn" ("string")) -> (w908:string)
              n304 = call "BaseProcess.get i attribute.vi"("i ref in"=w897, "error in (no error)"=w896) -> ("i ref out"=w895:refnum<vi>, "i attribute"=w905:T15, "error out"=w894:errorcluster)  [unwired: 15 in]
              n305 = Unbundle By Name(w905) -> ("Special"=w912:string[])
              n306 = call-poly "CoreLib.data 2 byte array.vi"("string"=w908) -> ("byteArray out"=w906:T1)  [unwired: 18 in]
              n307 = Index Array(array=w912, index=0) -> (element=w904:string)
              n308 = call-poly "CoreLib.data 2 byte array.vi"("byteArray"=w906, "f64"=w910) -> ("byteArray out"=w909:T1)  [unwired: 17 in]
              n309 = call "BaseProcess.call process 2.vi"("i ref in"=w895, "Object"=w904, "Selector"="SetValue", "Data Descriptor"="C:N;S:1;S:1", "Data"=w909, "error in (no error)"=w894) -> ("i ref out"=w892:refnum<vi>, "error out"=w893:errorcluster)  [unwired: 12 in]
            }
            frame Error {
              n310 = call "CoreLib.set data type mismatch.vi"("error in (no error)"=w915, "error source"=w913) -> ("error out"=w914:errorcluster)  [unwired: 17 in]
            }
          }
          n311 = call "BaseProcess.set event status.vi"("i ref in"=w879, "EventStatus"=w876, "error in (no error)"=w878) -> ("i ref out"=w875:refnum<vi>, "error out"=w877:errorcluster)  [unwired: 14 in, 1 out]
          n312 = case shown="Error" w877 {
            selector: w877 -> [_ w889]
            tunnel: [w886 w888] -> w880
            frame No Error {
              n313 = call-poly "CoreLib.data 2 byte array.vi"() -> ("byteArray out"=w886:T1)  [unwired: 19 in]
            }
            frame Error {
              n314 = Unbundle By Name(w889) -> ("source"=w887:string)
              n315 = call-poly "CoreLib.data 2 byte array.vi"("string"=w887) -> ("byteArray out"=w888:T1)  [unwired: 18 in]
            }
          }
          n316 = Unbundle By Name(w877) -> ("code"=w883:i32)
          n317 = Bundle By Name(cluster=w882, "Data"=w880, "Error #"=w883, "Data Descriptor"="D:1") -> (w881:T2)
        }
        frame "EmergencyOff" {
          n318 = call "PSChannelBase.get nof channels.vi"("i ref in"=w920, "error in (no error)"=w919) -> ("i ref out"=w923:refnum<vi>, "NofChannels"=w924:i32, "error out"=w922:errorcluster)  [unwired: 15 in]
          n319 = for {
            N: w924 -> [_]
            tunnel: [w942] -> w921 mode=indexing
            tunnel: [w941] -> w918
            tunnel: w923 -> [w937]
            tunnel: w922 -> [w936]
            i -> [w938]
            w935 = FALSE
            n320 = call "PSChannelBase.get channel names.vi"("i ref in"=w937, "channelIndex"=w938, "error in (no error)"=w936) -> ("i ref out"=w940:refnum<vi>, "logicalName"=w933:string, "error out"=w939:errorcluster)  [unwired: 13 in, 1 out]
            n321 = call "BaseProcess.get i attribute.vi"("i ref in"=w940, "error in (no error)"=w939) -> ("i ref out"=w951:refnum<vi>, "i attribute"=w954:T15, "error out"=w955:errorcluster)  [unwired: 15 in]
            n322 = Unbundle By Name(w954) -> ("Special"=w953:string[])
            n323 = Concatenate Strings(w933, "DOTOn" ("string")) -> (w944:string)
            n324 = Boolean To (0,1)(Boolean=w935) -> (0, 1=w934:i16)
            n325 = call-poly "CoreLib.data 2 byte array.vi"("string"=w944) -> ("byteArray out"=w947:T1)  [unwired: 18 in]
            n326 = Index Array(array=w953, index=0) -> (element=w950:string)
            n327 = call-poly "CoreLib.data 2 byte array.vi"("byteArray"=w947, "i16"=w934) -> ("byteArray out"=w946:T1)  [unwired: 17 in]
            n328 = call-poly "CoreLib.data 2 byte array.vi"("byteArray"=w946, "i16"=w934) -> ("byteArray out"=w945:T1)  [unwired: 17 in]
            n329 = call "BaseProcess.call process 2.vi"("i ref in"=w951, "Object"=w950, "Selector"="SetValue", "Data Descriptor"="C:N;S:1;S:1", "Data"=w945, "error in (no error)"=w955) -> ("i ref out"=w941:refnum<vi>, "error out"=w942:errorcluster)  [unwired: 12 in]
            n330 = Type Cast(x=w935) -> (*(type *) &x=w958:string)  [unwired: 1 in]
            n331 = call "PSChannelBase.update services and attribute data.vi"("i ref in"=w941, "direction"=PSChannelBase.directionType."update nominal value", "service"=PSChannelBase.serviceType."onOff", "value"=w958, "channelNumber"=w938) -> ()  [unwired: 12 in, 3 out]
          }
          n332 = Merge Errors(w921) -> (w917:errorcluster)
          n333 = call "BaseProcess.set event status.vi"("i ref in"=w918, "EventStatus"=w927, "error in (no error)"=w917) -> ("i ref out"=w926:refnum<vi>, "error out"=w928:errorcluster)  [unwired: 14 in, 1 out]
          n334 = case shown="Error" w928 {
            selector: w928 -> [_ w962]
            tunnel: [w959 w961] -> w929
            frame No Error {
              n335 = call-poly "CoreLib.data 2 byte array.vi"() -> ("byteArray out"=w959:T1)  [unwired: 19 in]
            }
            frame Error {
              n336 = Unbundle By Name(w962) -> ("source"=w960:string)
              n337 = call-poly "CoreLib.data 2 byte array.vi"("string"=w960) -> ("byteArray out"=w961:T1)  [unwired: 18 in]
            }
          }
          n338 = Unbundle By Name(w928) -> ("code"=w932:i32)
          n339 = Bundle By Name(cluster=w931, "Data"=w929, "Error #"=w932, "Data Descriptor"="D:1") -> (w930:T2)
        }
      }
      n340 = case "Default?" shown="False" w9 {
        tunnel: w11 -> [w19 _]
        tunnel: w10 -> [w18 _]
        frame False {
          n341 = call "DeviceBase.set device state.vi"("i ref in"=w18, "implicit"=TRUE, "device error"=w19) -> ()  [unwired: 14 in, 3 out]
        }
        frame True {
        }
      }
    }
    frame Error {
    }
  }
  "answer cluster" <- w7
  "i ref out" <- w3
  "error out" <- w2
